vi "equilibrium_measurements_autofocus_build.vi"() -> ()   [LabVIEW 2019]
uses:
  <vilib>/userDefined/High Color/IMAQdx.ctl
  <vilib>/vision/driver/IMAQdx.llb/IMAQdx Attribute Type.ctl
  <vilib>/vision/Management.llb/Cast Image 2 Method.ctl
  <vilib>/DAQmx/write.llb/DAQmx Write (Analog DBL 1Chan 1Samp).vi
  <vilib>/DAQmx/write.llb/DAQmx Write (Digital Bool 1Line 1Point).vi
  <vilib>/DAQmx/read.llb/DAQmx Read (Analog DBL 1Chan 1Samp).vi
  <vilib>/Analysis/baseanly.llb/Mean (DBL).vi
  <vilib>/DAQmx/create/channels.llb/DAQmx Create Channel (AO-Voltage-Basic).vi
  <vilib>/DAQmx/miscellaneous.llb/DAQmx Fill In Error Info.vi
  <vilib>/DAQmx/create/channels.llb/DAQmx Create Channel (AI-Temperature-Thermocouple).vi
  <vilib>/DAQmx/create/channels.llb/DAQmx Create Channel (DO-Digital Output).vi
  <vilib>/DAQmx/create/channels.llb/DAQmx Create Channel (CO-Pulse Generation-Frequency).vi
  <vilib>/DAQmx/configure/timing.llb/DAQmx Timing (Implicit).vi
  <vilib>/vision/driver/NI_Vision_Acquisition_Software.lvlib
  <resource>/objmgr/imaqdx.rc
  <vilib>/vision/NI_Vision_Development_Module.lvlib
  <vilib>/Analysis/NI_AALBase.lvlib
  <resource>/objmgr/daqmx.rc
panel:
  out "x-y":dbl
  out "Waveform Chart":dynamicdata(graph)
  out "Autofocus":bool
  out "Turn":bool
  out "displacement":i32
  out "steps":i32=1000
  out "Direction":bool
  in  "Direction Line":tag="Dev3/port1/line4"
  in  "Enable Drive":bool
  in  "Enable Line":tag="Dev3/port1/line1"
  in  "Step Signal \nOutput Line":tag="/Dev3/PFI2"
  in  "Step Pulse Train \nFrequency (Hz)":dbl=200.0 format="%.6f"
  out "Video":bool
  in  "Action":i32(listbox)
  out "meanIntensity":dbl[](array[numeric])
  out "varLaplacian":dbl[](array[numeric])
  out "mean":dbl
  out "variance":dbl
  out "Avg Intensity":dbl(graph)=4.716017316017316
  in  "Activate":bool
  out "Var of Laplacian":dbl(graph)=701.3672509340029
  in  "ROI":T1={"Global Rectangle"=[], "Contours"=[{"Contour Type"=0, "ROI Type"=3, "Points"=[231, 86, 235, 90]}, {"Contour Type"=0, "ROI Type"=3, "Points"=[193, 50, 270, 125]}]}
  in  "error in":errorcluster
  in  "File path for video":string="C:\\Users\\Aniket\\Desktop\\mCherry_calibration\\new_lens\\laser_calibration\\laser_and_heating\\"
  in  "Laser profile file path":path=path "C:/Users/Aniket/Desktop/mCherry_calibration/new_lens/laser_calibration/laser_profiles/new_profile.txt"
  in  "Trigger Laser":bool
  in  "Power Generator":refnum<visa-resource-name>="COM3"
  in  "Desired \nTemperature":dbl=20.0 format="%#_13g"
  in  "PID Control":bool
  in  "Image file path \n(Do not add specify file extension - set to png)":path=path "C:/Users/Aniket/Desktop/mCherry_calibration/new_lens/laser_calibration/laser_profiles.txt"
  out "Current \nTemperature":dbl format="%0.2f"
  out "?":dbl[](graph)=[37.63236695538445]
  out "error out 7":errorcluster
  out "error out 6":errorcluster
  out "error out 5":errorcluster
  out "Exposure Time":dbl
  in  "ON/OFF":bool
  out "error out 3":errorcluster
  in  "LED":dbl(slide) scale=0.0..10.0
  in  "Refresh":bool
  out "Record":bool
  out "Processed Frames per Second":dbl
  out "Acquired Frame Rate":dbl
  out "error out":errorcluster
  out "Camera Display":T2(plugin-control) caption="Image Out"
  in  "Frame Rate":dbl=20.0
  out "Attribute Information Array":T4(array[cluster])
  in  "Session In":T5="cam0"
  # "Spot motion"
  # "Stage motion"
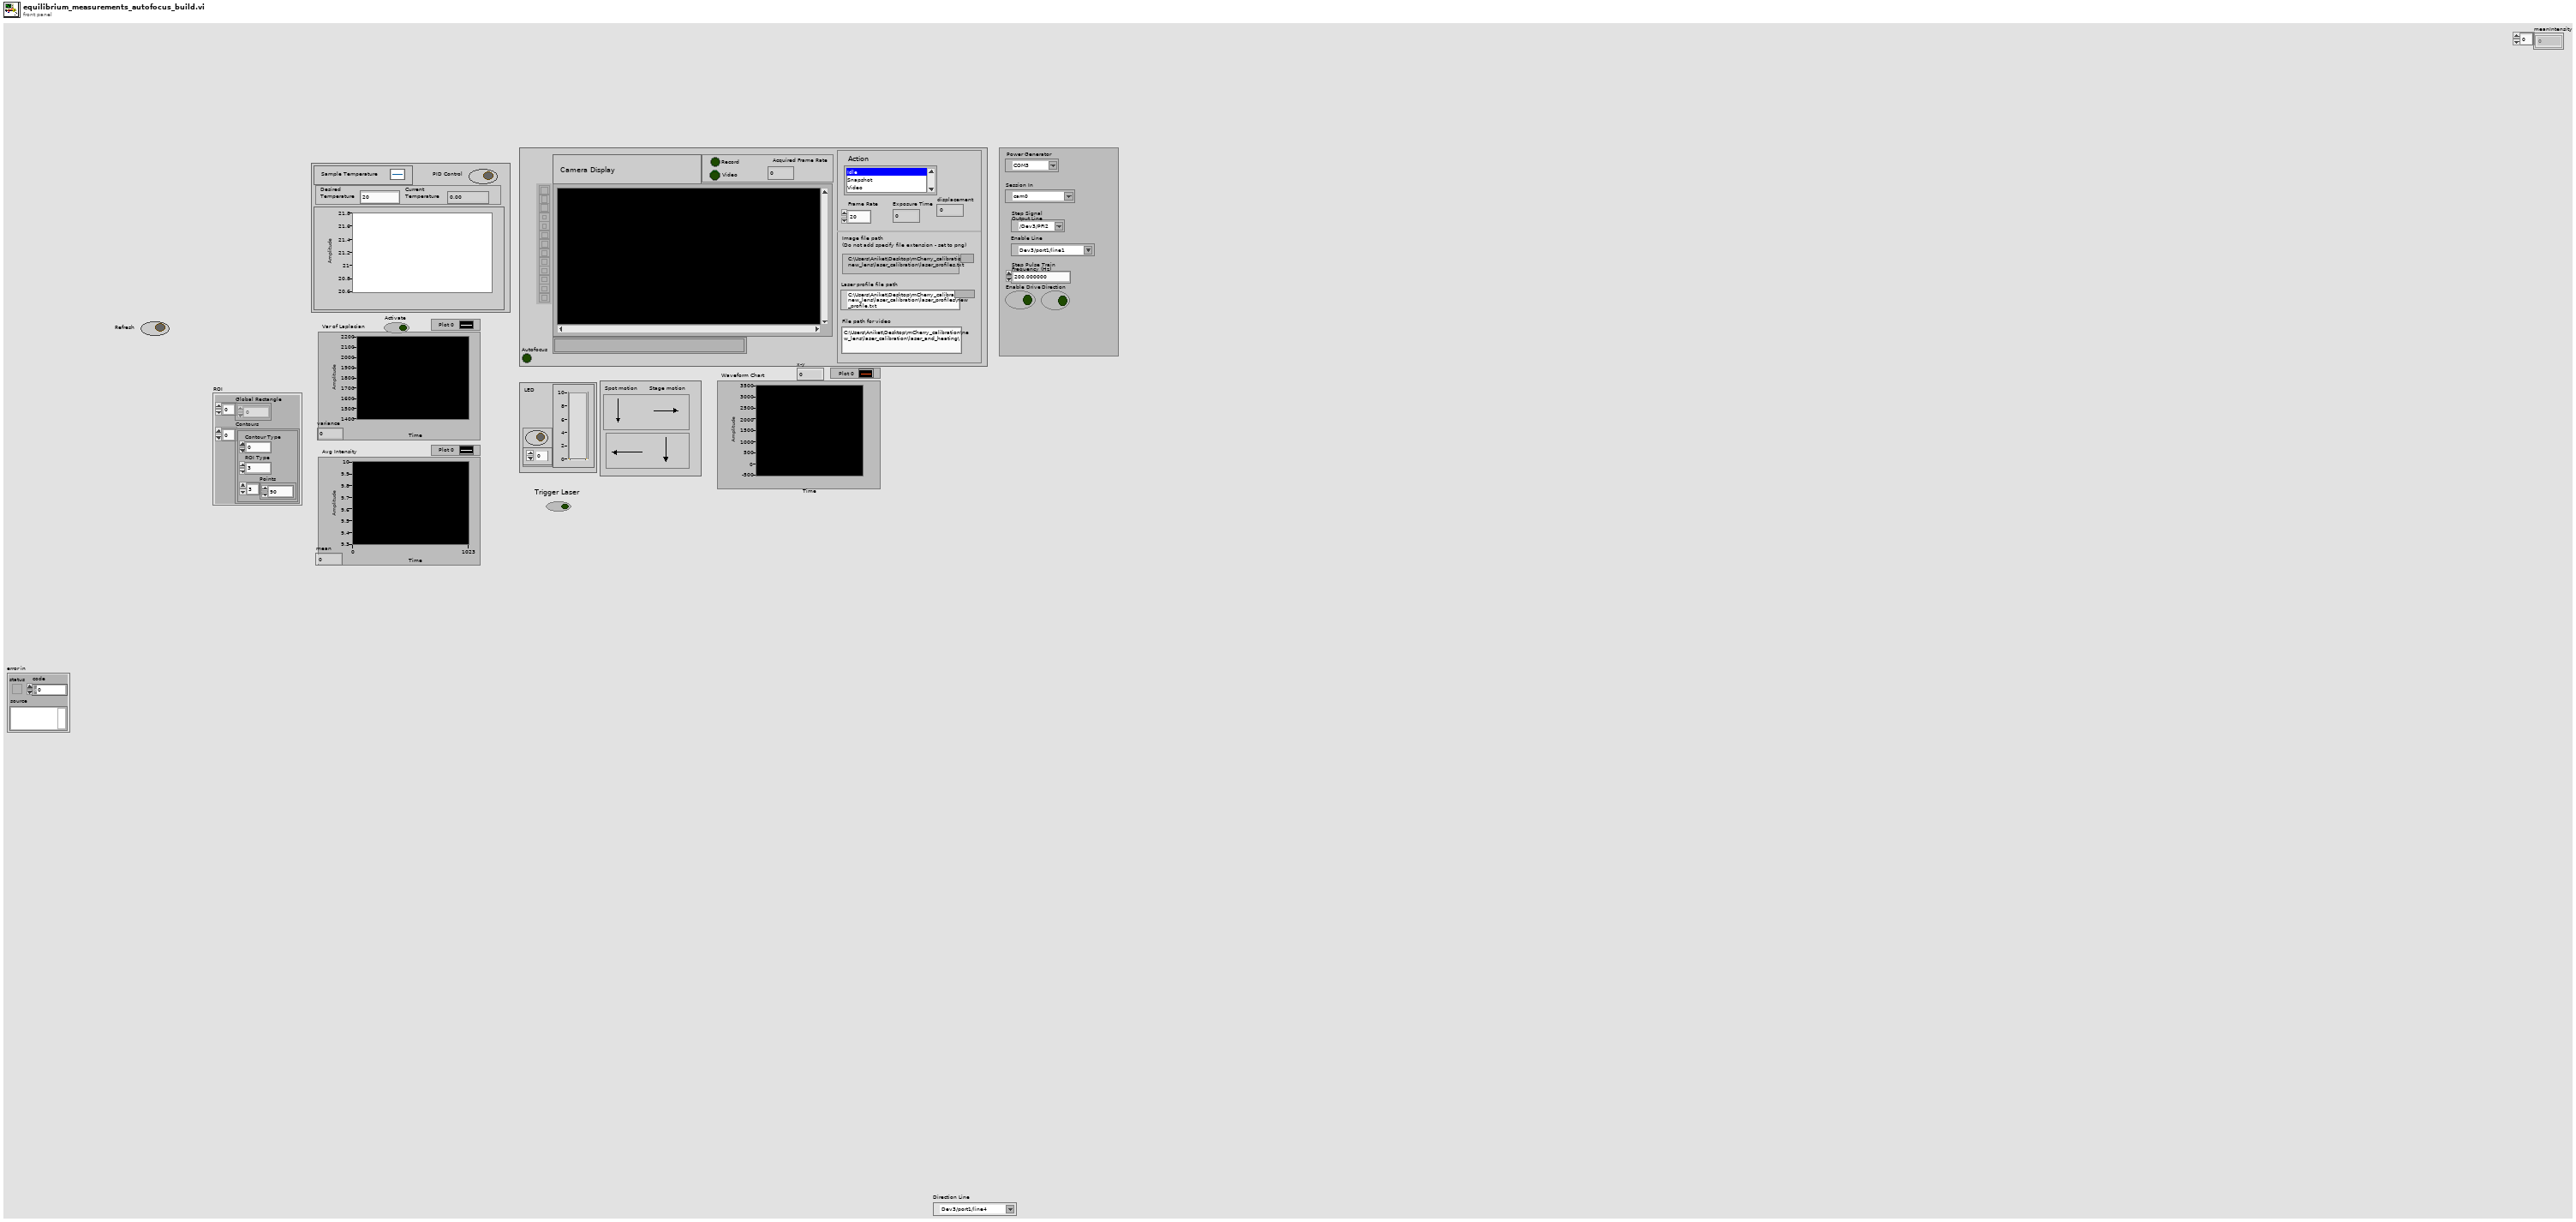
[diagram p1: front panel]
types:
  T1 = cluster{"Global Rectangle":i32[], "Contours":cluster{"Contour Type":u32, "ROI Type":u32, "Points":i32[]}[]}
  T2 = typedef "IMAQ Image.ctl" = refnum<image>
  T3 = typedef "NI_Vision_Acquisition_Software.lvlib/IMAQdx Attribute Type.ctl" = enum32{"U32", "I64", "DBL", "String", "Enum", "Bool", "Command"}
  T4 = cluster{"Attribute Type":T3, "Readable":bool, "Writable":bool, "Attribute Name":string}[]
  T5 = typedef "IMAQdx.ctl" = refnum<k21>
  T6 = typedef "Image Type" = u32
  T7 = typedef "ROI Descriptor" = cluster{"Global Rectangle":i32[], "Contours":cluster{"ID":enum32{"External", "Internal"}, "Type":u32, "Coordinates":i32[]}[]}
  T8 = typedef "IMAQ Rectangle" = cluster{"Left":i32, "Top":i32, "Right":i32, "Bottom":i32, "Rotation":dbl}
  T9 = cluster{"Mean Intensity":sgl, "Standard  Deviation":sgl, "Minimum Intensity":sgl, "Maximum Intensity":sgl}
  T10 = typedef "Cast Image 2 Method.ctl" = u32
  T11 = typedef "IMAQ AVI2 Refnum.ctl" = refnum<k20>
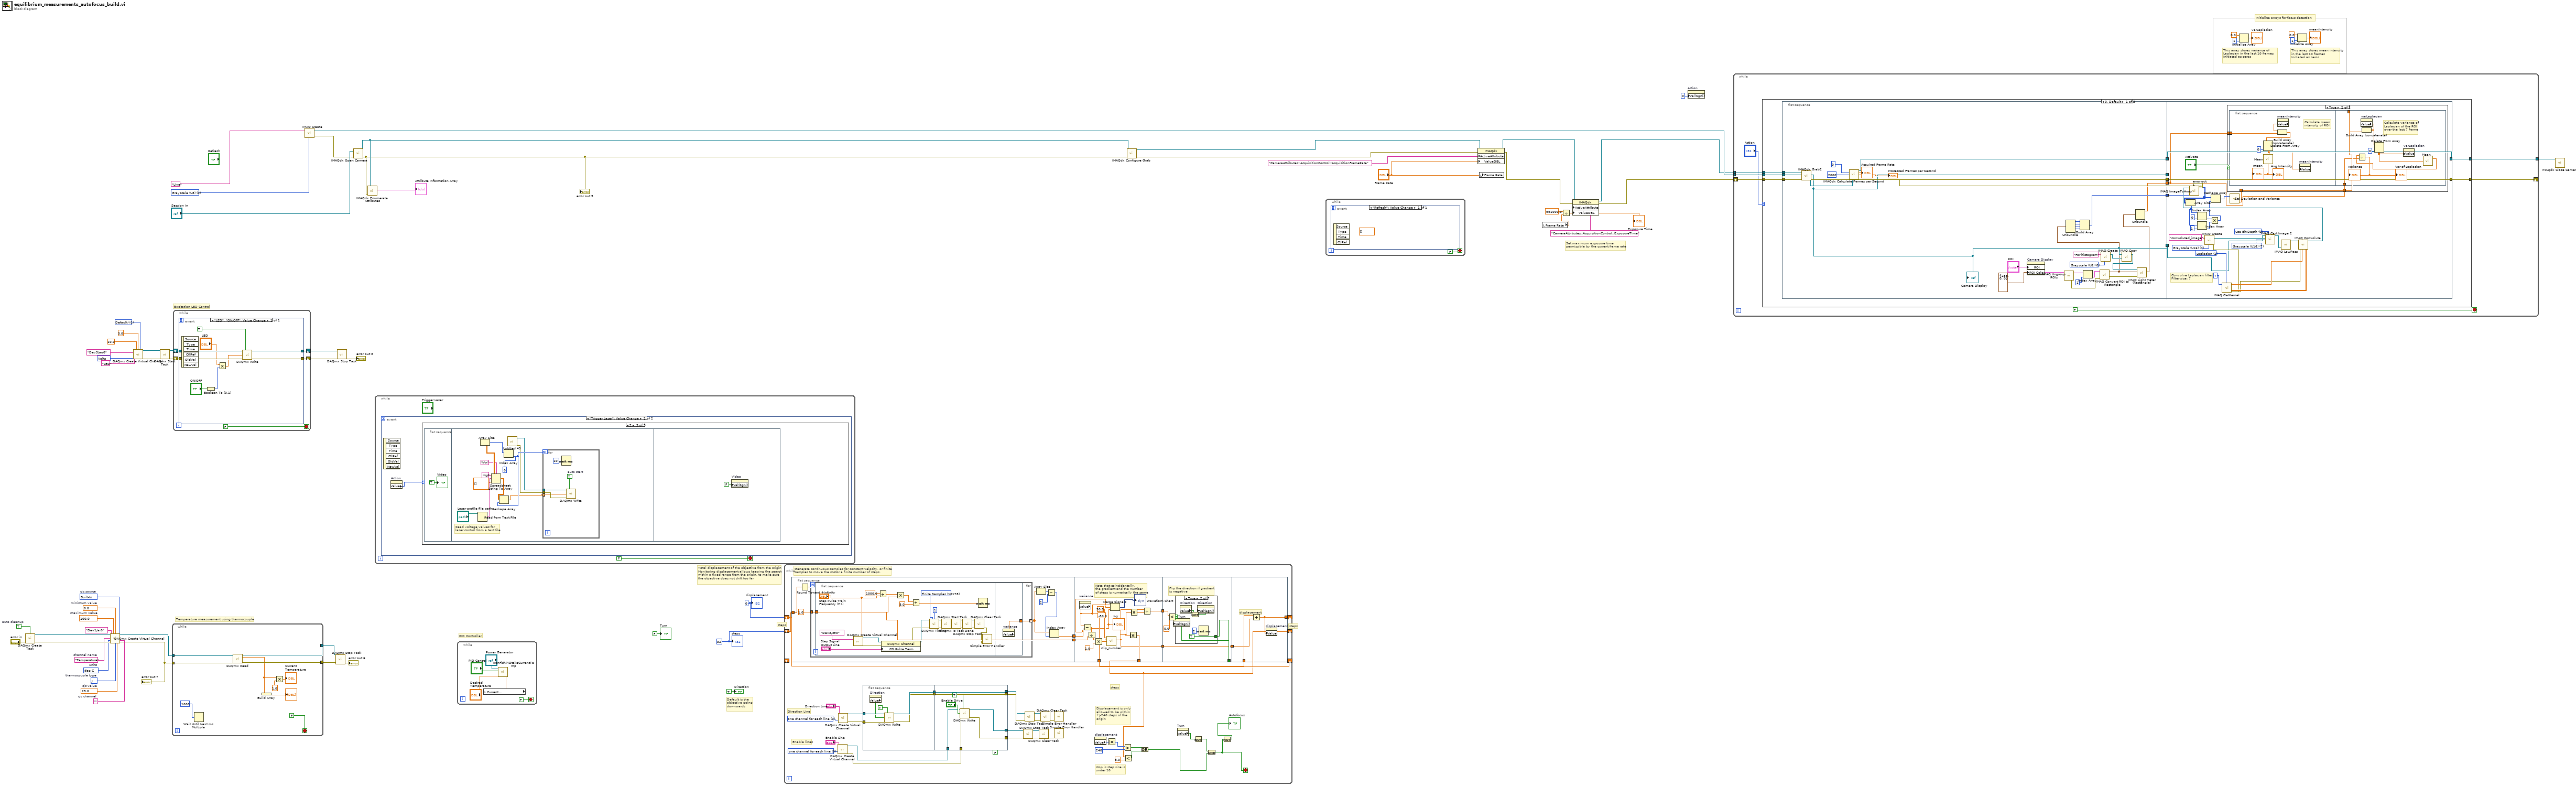
[diagram p0: block diagram]
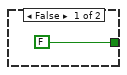
[diagram p2: hidden frame]
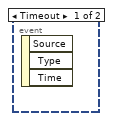
[diagram p3: hidden frame]
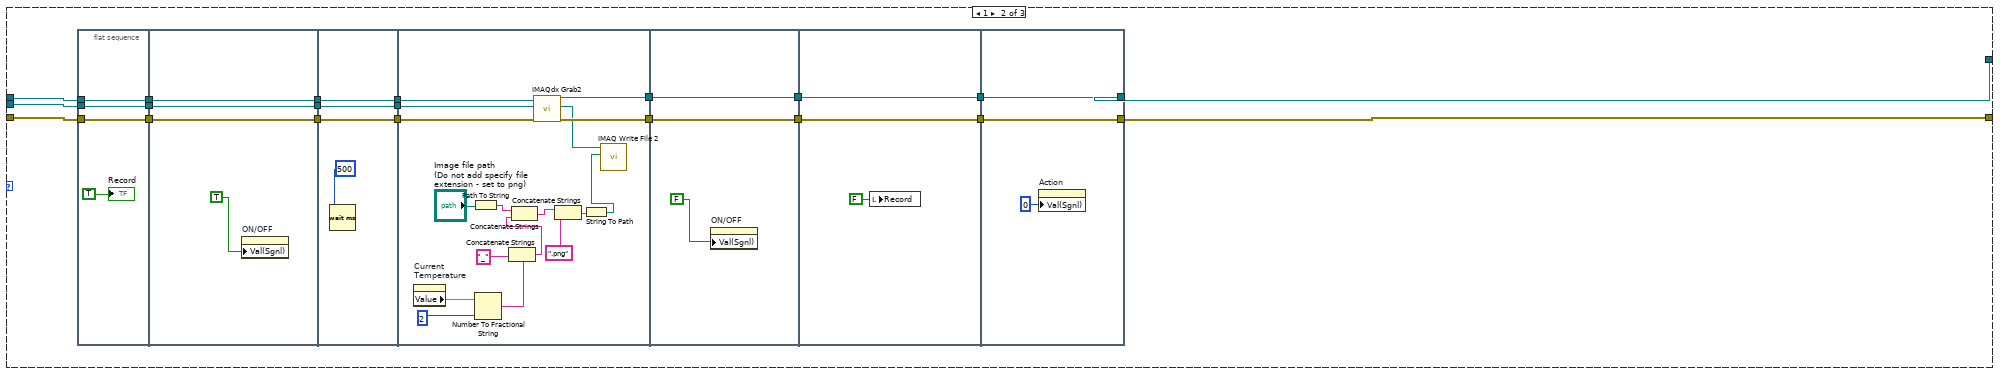
[diagram p7: hidden frame]
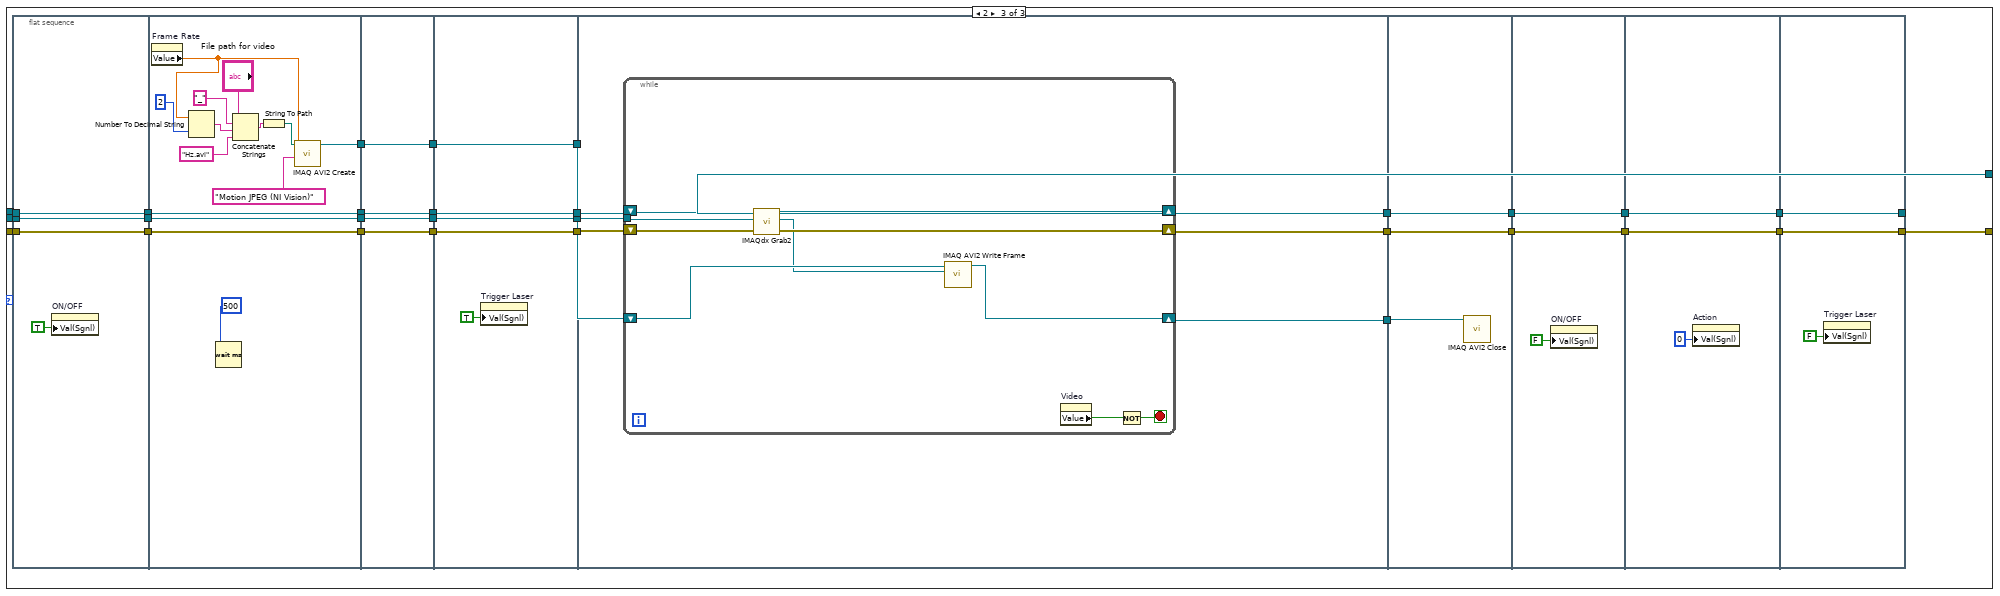
[diagram p8: hidden frame]
diagram:
  w4 = 0
  w3 = 32 ("samples per channel")
  w16 = 10200 items=["Built-In"=10200, "Constant Value"=10116, "Channel"=10113]  # cjc source
  w18 = ""  # cjc channel
  w19 = 25.0  # cjc value
  w20 = 10072 items=["J"=10072, "K"=10073, "N"=10077, "R"=10082, "S"=10085, "T"=10086, "B"=10047, "E"=10055]  # thermocouple type
  w21 = 10143 items=["deg C"=10143, "deg F"=10144, "Kelvins"=10325, "deg R"=10145, "From Custom Scale"=10065]  # units
  w17 = "Temperature"  # channel name
  w22 = 0.0  # minimum value
  w23 = 100.0  # maximum value
  w25 = TRUE  # auto cleanup
  w48 = 10348 items=["Volts"=10348, "From Custom Scale"=10065] ("units")
  w50 = -1 items=["Default"=-1, "RSE"=10083, "NRSE"=10078, "Differential"=10106, "Pseudodifferential"=12529] ("input terminal configuration")
  w62 = T6 0 items=["Grayscale (U8)", "Grayscale (I16)", "Grayscale (SGL)", "Complex (CSG)", "RGB (U32)", "HSL (U32)", "RGB (U64)", "Grayscale (U16)"] ("Image Type")
  # "Default is the\nobjective going\ndownwards"
  # "displacement"
  # "steps"
  # "steps"
  # "Total displacement of the objective from the origin\nMonitoring displacement allows keeping the search\nwithin a fixed range from the origin, to make sure\nthe objective does not drift too far"
  # "Set maximum exposure time \npermissible by the current frame rate"
  # "Excitation LED Control"
  # "Temperature measurement using thermocouple"
  # "PID Controller"
  # "Initialize arrays for focus detection"
  # "This array stores mean intensity in the last 10 frames\nInitiated as zeros"
  # "This array stores variance of Laplacian in the last 10 frames\nInitiated as zeros"
  n1 = call <vilib>:"DAQmx Create Task.vi"("auto cleanup"=w25, "error in"="error in") -> ("task out"=w24:refnum<k21>, "error out"=w26:errorcluster)  [unwired: 12 in]
  n2 = call-poly <vilib>:"DAQmx Create Virtual Channel.vi"("task in"=w24, "maximum value"=w23, "minimum value"=w22, "physical channels"=tag "Dev1/ai0", "cjc source"=w16, "name to assign"=w17, "units"=w21, "cjc channel"=w18, "error in"=w26, "thermocouple type"=w20, "cjc value"=w19) -> ("task out"=w15:refnum<k21>, "error out"=w14:errorcluster)  [unwired: 3 in]
  "error out 7" <- w14
  n3 = call-poly <vilib>:"DAQmx Create Virtual Channel.vi"("maximum value"=10.0, "minimum value"=0.0, "output terminal configuration"=w50, "physical channels"=tag "Dev3/ao0", "name to assign"="LED", "units"=w48) -> ("task out"=w46:refnum<k21>, "error out"=w45:errorcluster)  [unwired: 8 in]
  n4 = call <vilib>:"DAQmx Start Task.vi"("task/channels in"=w46, "error in"=w45) -> ("task out"=w44:refnum<k21>, "error out"=w43:errorcluster)  [unwired: 12 in]
  n5 = while {
    tunnel: w15 -> [w73]
    tunnel: w14 -> [w72]
    tunnel: [w71] -> w30
    tunnel: [w70] -> w29
    stop <- FALSE ("Monitor Temperature") stop-if-true
    n6 = Wait Until Next ms Multiple(millisecond multiple=u32 1000 ("millisecond timer value")) -> ()  [unwired: 1 out]
    n7 = call-poly <vilib>:"DAQmx Read.vi"("task/channels in"=w73, "error in"=w72) -> ("task out"=w71:refnum<k21>, "data"=w66:dbl, "error out"=w70:errorcluster)  [unwired: 11 in]
    n8 = Build Array(w66) -> (→"?":dbl[])
    n9 = Multiply(x=w66, y=1.0) -> (x*y=→"Current \nTemperature":dbl)
  }
  n10 = while {
    shift-right: [w77] -> w42
    shift-left: w44 -> [w79]
    shift-right: [w76] -> w41
    shift-left: w43 -> [w78]
    stop <- FALSE stop-if-true
    n11 = event shown="[0] \"LED\", \"ON/OFF\": Value Change" {
      selector: _ -> [_]
      dyn-events: _ -> [_]
      timeout: _ -> [_]
      tunnel: w79 -> [w88]
      tunnel: w78 -> [w87]
      tunnel: [w86] -> w77
      tunnel: [w85] -> w76
      event "LED", "ON/OFF": Value Change {
        n12 = event-data() -> ()  [unwired: 1 in, 6 out]
        n13 = Boolean To (0,1)(Boolean="ON/OFF") -> (0, 1=w81:i16)
        n14 = Multiply(x="LED", y=w81) -> (x*y=w80:dbl)
        n15 = call-poly <vilib>:"DAQmx Write.vi"("task/channels in"=w88, "auto start"=TRUE, "data"=w80, "error in"=w87) -> ("task out"=w86:refnum<k21>, "error out"=w85:errorcluster)  [unwired: 9 in, 1 out]
      }
    }
  }
  n16 = call "IMAQ Create"("Image Name"="Live", "Image Type"=w62) -> ("New Image"=w56:T2, "error out"=w55:errorcluster)  [unwired: 3 in]
  n17 = call <vilib>:"DAQmx Stop Task.vi"("task/channels in"=w30, "error in"=w29) -> ("error out"=→"error out 6":errorcluster)  [unwired: 12 in, 1 out]
  n18 = call <vilib>:"DAQmx Stop Task.vi"("task/channels in"=w42, "error in"=w41) -> ("error out"=→"error out 3":errorcluster)  [unwired: 12 in, 1 out]
  n19 = call <vilib>:"IMAQdx Open Camera.vi"("error in"=w55, "Session In"="Session In") -> ("error out"=w60:errorcluster, "Session Out"=w61:T5)  [unwired: 8 in]
  "error out 5" <- w60
  n20 = call <vilib>:"IMAQdx Enumerate Attributes.vi"("error in"=w60, "Session In"=w61) -> ("Attribute Information Array"=→"Attribute Information Array":T4)  [unwired: 7 in, 2 out]
  n21 = while {
    stop <- FALSE stop-if-true
    n22 = event shown="[1] \"Trigger Laser\": Value Change" {
      selector: _ -> [_ _]
      dyn-events: _ -> [_ _]
      timeout: _ -> [_ _]
      event Timeout {
        n23 = event-data() -> ()  [unwired: 1 in, 3 out]
      }
      event "Trigger Laser": Value Change {
        n24 = event-data() -> ()  [unwired: 1 in, 6 out]
        n25 = property on="Action" class="LstBox (strict)"() -> ("Value"=w90:i32)  [unwired: 2 in, 2 out]
        n26 = case shown="2" w90 {
          frame 0, Default {
          }
          frame 1 {
          }
          frame 2 {
            n27 = flat-sequence {
              frame #0 {
                "Video" <- TRUE ("Video")
              }
              frame #1 {
                # "Read voltage values for\nlaser control from a text file"
                n28 = Read from Text File(file (use dialog)="Laser profile file path") -> (text=w99:string)  [unwired: 3 in, 3 out]
                n29 = Spreadsheet String To Array(delimiter (Tab)="\r\n", format string="%f", spreadsheet string=w99, array type (2D Dbl)=dbl[][] []) -> (array=w101:dbl[][])
                n30 = Array Size(array=w101) -> (size(s)=w100:i32[])
                n31 = Index Array(array=w100, index=0) -> (element=w103:i32)
                n32 = Reshape Array(w101, w103) -> (w102:dbl[])
                n33 = call "Untitled 43.vi"() -> ("error out"=w92:errorcluster, "task out"=w93:refnum<k21>)  [unwired: 10 in]
                n34 = for {
                  N: w103 -> [_]
                  tunnel: w102 -> [w104] mode=indexing
                  tunnel: w93 -> [w106]
                  tunnel: w92 -> [w105]
                  w107 = TRUE  # auto start
                  n35 = Wait (ms)(milliseconds to wait=u32 10) -> ()  [unwired: 1 out]
                  n36 = call-poly <vilib>:"DAQmx Write.vi"("task/channels in"=w106, "auto start"=w107, "data"=w104, "error in"=w105) -> ()  [unwired: 9 in, 3 out]
                }
              }
              frame #2 {
                n37 = property on="Video" class="Bool (strict)"("Val(Sgnl)"=FALSE ("Value (Signaling)")) -> ()  [unwired: 2 in, 2 out]
              }
            }
          }
        }
      }
    }
  }
  n38 = while {
    stop <- FALSE stop-if-true
    n39 = local read "Current \nTemperature"() -> (w113:dbl)
    n40 = call "IronFishPIDtakeCurrentTemp.vi"(0:"Power Generator", "Switch"="PID Control", "Desired Temp"="Desired \nTemperature", "Current Temp"=w113) -> ()  [unwired: 4 in, 1 out]
  }
  n41 = while {
    shift-right: [w136] -> _
    shift-left: _ -> [_]
    shift-right: [w135] -> _
    shift-left: w4 -> [w134]
    shift-right: [w123] -> _
    shift-left: w3 -> [w133]
    stop <- w116 stop-if-true
    (unwired) FALSE
    w138 = 0 items=["one channel for each line", "one channel for all lines"] ("line grouping")
    w137 = 0 items=["one channel for each line", "one channel for all lines"] ("line grouping")
    # "stop is step size is \nunder 10"
    # "steps"
    # "Displacement is only\nallowed to be within \n+/-240 steps of the\norigin"
    # "Direction Line"
    # "Enable lines"
    # "Generate continuous samples for constant velocity, or finite \nsamples to move the motor a finite number of steps."
    n42 = flat-sequence {
      tunnel: [w178] -> w132
      tunnel: w133 -> [w172]
      tunnel: [w173] -> w117
      tunnel: [w209] -> w136
      tunnel: [w216] -> w123
      tunnel: w132 -> [w219]
      tunnel: [w217] -> w124
      tunnel: [w215] -> w122
      tunnel: w117 -> [w208]
      tunnel: [w224] -> w125
      tunnel: w124 -> [w222]
      tunnel: w122 -> [w224]
      tunnel: [w220] -> w121
      tunnel: w125 -> [w232]
      tunnel: [w231] -> w135
      tunnel: w134 -> [w230]
      frame #0 {
        w178 = 1.0 ("samples per channel")
        n43 = Round Toward +Infinity(x=w172) -> (ceil(x): smallest int >= x=w171:dbl)
        n44 = for {
          N: w171 -> [_]
          tunnel: w178 -> [w180]
          tunnel: [w179] -> w177 mode=indexing
          n45 = flat-sequence {
            tunnel: w180 -> [w200]
            tunnel: [w205] -> w179
            frame #0 {
              w194 = 10178 items=["Finite Samples"=10178, "Continuous Samples"=10123, "Hardware Timed Single Point"=12522] ("sample mode")
              n46 = call-poly <vilib>:"DAQmx Create Virtual Channel.vi"("frequency"="Step Pulse Train \nFrequency (Hz)", "counter"=tag "Dev3/ctr0") -> ("task out"=w186:refnum<k21>, "error out"=w185:errorcluster)  [unwired: 12 in]
              n47 = Divide(x=1000.0, y="Step Pulse Train \nFrequency (Hz)") -> (x/y=w189:dbl)
              n48 = property class="DAQmx Channel"(reference=w186, error in=w185, "CO.Pulse.Term"="Step Signal \nOutput Line") -> (reference out=w193:refnum<k21>, error out=w192:errorcluster)
              n49 = Multiply(x=w189, y=w200) -> (x*y=w191:dbl)
              n50 = Add(x=w191, y=5.0) -> (x+y=w197:dbl)
              n51 = call-poly <vilib>:"DAQmx Timing.vi"("task/channels in"=w193, "sample mode"=w194, "samples per channel"=1, "error in"=w192) -> ("task out"=w196:refnum<k21>, "error out"=w195:errorcluster)  [unwired: 10 in]
              n52 = call <vilib>:"DAQmx Start Task.vi"("task/channels in"=w196, "error in"=w195) -> ("task out"=w199:refnum<k21>, "error out"=w198:errorcluster)  [unwired: 12 in]
              n53 = call <vilib>:"DAQmx Is Task Done.vi"("task/channels in"=w199, "error in"=w198) -> ("task out"=w203:refnum<k21>, "error out"=w202:errorcluster)  [unwired: 11 in, 1 out]
              n54 = call <vilib>:"DAQmx Stop Task.vi"("task/channels in"=w203, "error in"=w202) -> ("task out"=w204:refnum<k21>, "error out"=w201:errorcluster)  [unwired: 12 in]
              n55 = call <vilib>:"DAQmx Clear Task.vi"("task in"=w204, "error in"=w201) -> ("error out"=w181:errorcluster)  [unwired: 13 in]
              n56 = Wait (ms)(milliseconds to wait=w197) -> ()  [unwired: 1 out]
              n57 = call <vilib>:"Simple Error Handler.vi"("error in (no error)"=w181) -> ()  [unwired: 4 in, 5 out]
            }
            frame #1 {
              n58 = property on="variance" class="DigNum (strict)"() -> ("Value"=w205:dbl)  [unwired: 2 in, 2 out]
            }
          }
        }
        n59 = Array Size(array=w177) -> (size(s)=w176:i32)
        n60 = Subtract(x=w176, y=2) -> (x-y=w174:i32)
        n61 = Index Array(array=w177, index=w174) -> (element=w173:dbl)
      }
      frame #1 {
        # "Note that coincidentally,\nthe gradient and the number\nof steps is numerically the same"
        n62 = property on="variance" class="DigNum (strict)"() -> ("Value"=w209:dbl)  [unwired: 2 in, 2 out]
        n63 = Subtract(x=w209, y=w208) -> (x-y=w207:dbl)
        "x-y" <- w207
        n64 = Divide(x=w207, y=w219) -> (x/y=w211:dbl)
        n65 = Multiply(x=w211, y=1.0) -> (x*y=w212:dbl)
        n66 = call "clip_number.vi"("x"=w212, "lower limit"=-50.0, "upper limit"=50.0) -> ("x-y"=w215:dbl)  [unwired: 8 in]
        n67 = Merge Signals(w209, w208, w207) -> (→"Waveform Chart":dynamicdata)
        n68 = Absolute Value(x=w215) -> (abs(x)=w216:dbl)
        n69 = Absolute Value(x=w215) -> (abs(x)=w218:dbl)
        n70 = Divide(x=w215, y=w218) -> (x/y=w217:dbl)
      }
      frame #2 {
        # "Flip the direction if gradient\nis negative"
        n71 = Less?(x=w222, y=0.0) -> (x < y?=w223:bool)
        n72 = case shown="True" w223 {
          tunnel: [FALSE ("Value (Signaling)") TRUE ("Value (Signaling)")] -> w220
          frame False {
          }
          frame True {
            n73 = property on="Direction" class="Bool (strict)"() -> ("Value"=w229:bool)  [unwired: 2 in, 2 out]
            n74 = Not(x=w229) -> (.not. x?=w228:bool)
            n75 = property on="Direction" class="Bool (strict)"("Val(Sgnl)"=w228) -> ()  [unwired: 2 in, 2 out]
            n76 = Wait (ms)(milliseconds to wait=u32 2) -> ()  [unwired: 1 out]
          }
        }
      }
      frame #3 {
        n77 = Add(x=w230, y=w232) -> (x+y=w231:dbl)
        n78 = property on="displacement" class="DigNum (strict)"("Value"=w231) -> ()  [unwired: 2 in, 2 out]
      }
    }
    n79 = call-poly <vilib>:"DAQmx Create Virtual Channel.vi"("lines"="Enable Line", "line grouping"=w137) -> ("task out"=w151:refnum<k21>, "error out"=w152:errorcluster)  [unwired: 12 in]
    n80 = call-poly <vilib>:"DAQmx Create Virtual Channel.vi"("lines"="Direction Line", "line grouping"=w138) -> ("task out"=w147:refnum<k21>, "error out"=w148:errorcluster)  [unwired: 12 in]
    n81 = flat-sequence {
      tunnel: w147 -> [w161]
      tunnel: w148 -> [w160]
      tunnel: [w159] -> w156
      tunnel: [w158] -> w155
      tunnel: [w169] -> w150
      tunnel: [w170] -> w149
      tunnel: w156 -> [w170]
      tunnel: w155 -> [w169]
      tunnel: w151 -> [w166]
      tunnel: w152 -> [w165]
      tunnel: [w164] -> w153
      tunnel: [w163] -> w154
      frame #0 {
        n82 = property on="Direction" class="Bool (strict)"() -> ("Value"=w157:bool)  [unwired: 2 in, 2 out]
        n83 = call-poly <vilib>:"DAQmx Write.vi"("task/channels in"=w161, "auto start"=TRUE, "data"=w157, "error in"=w160) -> ("task out"=w159:refnum<k21>, "error out"=w158:errorcluster)  [unwired: 9 in, 1 out]
      }
      frame #1 {
        n84 = call-poly <vilib>:"DAQmx Write.vi"("task/channels in"=w166, "auto start"=TRUE, "data"="Enable Drive", "error in"=w165) -> ("task out"=w164:refnum<k21>, "error out"=w163:errorcluster)  [unwired: 9 in, 1 out]
      }
    }
    n85 = call <vilib>:"DAQmx Stop Task.vi"("task/channels in"=w153, "error in"=w154) -> ("task out"=w140:refnum<k21>, "error out"=w141:errorcluster)  [unwired: 12 in]
    n86 = call <vilib>:"DAQmx Stop Task.vi"("task/channels in"=w149, "error in"=w150) -> ("task out"=w146:refnum<k21>, "error out"=w145:errorcluster)  [unwired: 12 in]
    n87 = call <vilib>:"DAQmx Clear Task.vi"("task in"=w140, "error in"=w141) -> ("error out"=w142:errorcluster)  [unwired: 13 in]
    n88 = call <vilib>:"DAQmx Clear Task.vi"("task in"=w146, "error in"=w145) -> ("error out"=w144:errorcluster)  [unwired: 13 in]
    n89 = call <vilib>:"Simple Error Handler.vi"("error in (no error)"=w144) -> ()  [unwired: 4 in, 5 out]
    n90 = call <vilib>:"Simple Error Handler.vi"("error in (no error)"=w142) -> ()  [unwired: 4 in, 5 out]
    n91 = property on="displacement" class="DigNum (strict)"() -> ("Value"=w130:i32)  [unwired: 2 in, 2 out]
    n92 = Absolute Value(x=w130) -> (abs(x)=w129:i32)
    n93 = Greater?(x=w129, y=240) -> (0:w128:bool)
    n94 = Less?(x=w123, y=8.0) -> (x < y?=w127:bool)
    n95 = Or(x=w128, y=w127) -> (x .or. y?=w118:bool)
    n96 = property on="Turn" class="Bool (strict)"("Val(Sgnl)"=w121) -> ()  [unwired: 2 in, 2 out]
    n97 = property on="Turn" class="Bool (strict)"() -> ("Value"=w120:bool)  [unwired: 2 in, 2 out]
    n98 = Not(x=w120) -> (.not. x?=w119:bool)
    n99 = And(x=w119, y=w118) -> (x .and. y?=w116:bool)
    n100 = Not(x=w116) -> (.not. x?=→"Autofocus":bool)
  }
  n101 = call <vilib>:"IMAQdx Configure Grab.vi"("error in"=w60, "Session In"=w61) -> ("error out"=w58:errorcluster, "Session Out"=w39:T5)  [unwired: 8 in]
  n102 = while {
    stop <- FALSE stop-if-true
    n103 = event shown="[0] \"Refresh\": Value Change" {
      selector: _ -> [_]
      dyn-events: _ -> [_]
      timeout: _ -> [_]
      event "Refresh": Value Change {
        (unwired) dbl[] [] ("History Data")
        n104 = event-data() -> ()  [unwired: 1 in, 4 out]
      }
    }
  }
  n105 = property class="IMAQdx"(reference=w39, error in=w58, "ActiveAttribute"="CameraAttributes::AcquisitionControl::AcquisitionFrameRate", "ValueDBL"="Frame Rate") -> (reference out=w34:T5, error out=w32:errorcluster)
  n106 = local write "Frame Rate"("Frame Rate") -> ()
  n107 = local read "Frame Rate"() -> (w36:dbl)
  n108 = Divide(x=991000.0, y=w36) -> (x/y=w35:dbl)
  "Exposure Time" <- w35
  n109 = property class="IMAQdx"(reference=w34, error in=w32, "ActiveAttribute"="CameraAttributes::AcquisitionControl::ExposureTime", "ValueDBL"=w35) -> (reference out=w33:T5, error out=w31:errorcluster)
  n110 = property on="Action" class="LstBox (strict)"("Val(Sgnl)"=0 ("Value (Signaling)")) -> ()  [unwired: 2 in, 2 out]
  n111 = while {
    tunnel: w33 -> [w240]
    tunnel: w56 -> [w238]
    shift-right: [w237] -> w54
    shift-left: w31 -> [w239]
    tunnel: [w234] -> w6
    stop <- FALSE ("Stop") stop-if-true
    n112 = case shown="0, Default" "Action" {
      tunnel: w240 -> [w251 w343 w414]
      tunnel: w239 -> [w250 w345 w412]
      tunnel: w238 -> [w249 w344 w413]
      tunnel: [w248 w346 w410] -> w237
      tunnel: [w247 w347 w411] -> w234
      frame 0, Default {
        n113 = flat-sequence {
          tunnel: w251 -> [w281]
          tunnel: w250 -> [w280]
          tunnel: w249 -> [w279]
          tunnel: [w278] -> w246
          tunnel: [w276] -> w245
          tunnel: [w263] -> w244
          tunnel: [w263] -> w243
          tunnel: [w255] -> w242
          tunnel: [w252] -> w241
          tunnel: [w309] -> w247
          tunnel: [w310] -> w248
          tunnel: w246 -> [w310]
          tunnel: w245 -> [w309]
          tunnel: w244 -> [_]
          tunnel: w243 -> [w291]
          tunnel: w242 -> [w300]
          tunnel: w241 -> [w282]
          frame #0 {
            w264 = T6 0 items=["Grayscale (U8)", "Grayscale (I16)", "Grayscale (SGL)", "Complex (CSG)", "RGB (U32)", "HSL (U32)", "RGB (U64)", "Grayscale (U16)"] ("Image Type")
            n114 = call <vilib>:"IMAQdx Grab2.vi"("error in"=w280, "Image In"=w279, "Session In"=w281) -> ("error out"=w278:errorcluster, "Image Out"=w263:T2, "Session Out"=w277:T5)  [unwired: 5 in, 1 out]
            "Camera Display" <- w263
            n115 = call <vilib>:"IMAQdx Calculate Frames per Second.vi"("Session In"=w277, "Buffer Number"=u32 0, "Minimum Display Update Interval (ms)"=u32 2000) -> ("Session Out"=w276:T5, "Acquired Frames per Second"=→"Acquired Frame Rate":dbl, "Processed Frames per Second"=→"Processed Frames per Second":dbl)  [unwired: 6 in, 4 out]
            n116 = property on="Camera Display" class="ImageControl"("ROI"="ROI", "ROI Color"=cluster{"Red":u8, "Green":u8, "Blue":u8} {"Red"=255, "Green"=0, "Blue"=0}) -> ()  [unwired: 2 in, 2 out]
            n117 = call "IMAQ Ungroup ROIs"("ROI Descriptor"="ROI") -> ("error out"=w267:errorcluster, "ROI Descriptors out"=w270:T7[])  [unwired: 3 in]
            n118 = Index Array(array=w270, index=1) -> (element=w268:T7)
            n119 = call "IMAQ Convert ROI to Rectangle"("error in (no error)"=w267, "ROI Descriptor"=w268) -> ("error out"=w266:errorcluster, "Rectangle"=w260:T8)  [unwired: 7 in]
            n120 = Unbundle(w260) -> ("Left"=w259:i32, "Top"=w258:i32, "Right"=w257:i32, "Bottom"=w256:i32)  [unwired: 1 out]
            n121 = Build Array(w259, w258, w257, w256) -> (w255:i32[])
            n122 = call "IMAQ Create"("Image Name"="For histogram", "Image Type"=w264) -> ("New Image"=w262:T2)  [unwired: 3 in, 1 out]
            n123 = call "IMAQ Copy"("Image Dst"=w262, "Image Src"=w263) -> ("Image Dst Out"=w261:T2)  [unwired: 4 in, 1 out]
            n124 = call "IMAQ Light Meter (Rectangle)"("error in (no error)"=w266, "Rectangle"=w260, "Image"=w261) -> ("Gray Level Intensities"=w253:T9)  [unwired: 4 in, 4 out]
            n125 = Unbundle(w253) -> ("Mean Intensity"=w252:sgl)  [unwired: 3 out]
          }
          frame #1 {
            w287 = T6 7 items=["Grayscale (U8)", "Grayscale (I16)", "Grayscale (SGL)", "Complex (CSG)", "RGB (U32)", "HSL (U32)", "RGB (U64)", "Grayscale (U16)"] ("Image Type")
            w290 = T10 0 items=["Use Bit Depth", "Shift", "Use Lookup Table"] ("Method")
            w305 = u16 2 items=["Gradient"=1, "Laplacian"=2, "Smoothing"=3, "Gaussian"=4] ("Kernel Family")
            w307 = T6 7 items=["Grayscale (U8)", "Grayscale (I16)", "Grayscale (SGL)", "Complex (CSG)", "RGB (U32)", "HSL (U32)", "RGB (U64)", "Grayscale (U16)"] ("Image Type")
            # "Convolve Laplacian filter \nFilter size: 7"
            n126 = call "IMAQ Create"("Image Name"="convoluted_image", "Image Type"=w307) -> ("New Image"=w289:T2, "error out"=w301:errorcluster)  [unwired: 3 in]
            n127 = call "IMAQ GetKernel"("Kernel Family"=w305, "error in (no error)"=w301, "Kernel Size (3,5,...)"=7) -> ("error out"=w302:errorcluster, "Kernel"=w303:sgl[][], "Divider"=w304:sgl)  [unwired: 5 in, 1 out]
            n128 = call "IMAQ Cast Image 2"("Image Src"=w291, "Method"=w290, "Image Dst"=w289, "Image Type"=w287) -> ("Image Dst Out"=w288:T2)  [unwired: 10 in, 1 out]
            n129 = call "IMAQ LowPass"("Image Src"=w288) -> ("Image Dst Out"=w292:T2)  [unwired: 6 in, 1 out]
            n130 = call "IMAQ Convolute"("Kernel"=w303, "Divider (kernel sum)"=w304, "error in (no error)"=w302, "Image Src"=w292) -> ("Image Dst Out"=w299:T2)  [unwired: 6 in, 1 out]
            n131 = call "IMAQ ImageToArray"("Optional Rectangle"=w300, "Image"=w299) -> ("Image Pixels (U16)"=w283:u16[][])  [unwired: 2 in, 4 out]
            n132 = Array Size(array=w283) -> (size(s)=w286:i32[])
            n133 = Index Array(array=w286, index=0 ("index (row)")) -> (element=w296:i32)
            n134 = Index Array(array=w286, index=1) -> (element=w295:i32)
            n135 = Multiply(x=w296, y=w295) -> (x*y=w285:i32)
            n136 = Reshape Array(w283, w285) -> (w284:u16[])
            n137 = call <vilib>:"Std Deviation and Variance.vi"("X"=w284) -> ("variance"=w293:dbl)  [unwired: 1 in, 2 out]
            n138 = case shown="True" "Activate" {
              tunnel: w293 -> [_ w313]
              tunnel: w282 -> [_ w312]
              tunnel: w282 -> [_ w311]
              frame False {
              }
              frame True {
                n139 = flat-sequence {
                  tunnel: w311 -> [w314]
                  tunnel: w313 -> [w323]
                  tunnel: w312 -> [w327]
                  frame #0 {
                    # "Calculate mean \nintensity of ROI"
                    n140 = property on="meanIntensity" class="Arr (strict)"() -> ("Value"=w317:dbl[])  [unwired: 2 in, 2 out]
                    n141 = Build Array (concatenate)(w317, w314) -> (w316:dbl[])
                    n142 = Delete From Array(array=w316, index=0) -> (array with subset deleted=w315:dbl[])  [unwired: 1 in, 1 out]
                    n143 = call-poly <vilib>:"Mean.vi"("X"=w315) -> ("mean"=→"Avg Intensity" →"mean":dbl)  [unwired: 1 out]
                    n144 = property on="meanIntensity" class="Arr (strict)"("Value"=w315) -> ()  [unwired: 2 in, 2 out]
                  }
                  frame #1 {
                    # "Calculate variance of\nLaplacian of the ROI\nover the last 7 frame"
                    n145 = property on="varLaplacian" class="Arr (strict)"() -> ("Value"=w324:dbl[])  [unwired: 2 in, 2 out]
                    n146 = Build Array (concatenate)(w324, w323) -> (w322:dbl[])
                    n147 = Delete From Array(array=w322, index=0) -> (array with subset deleted=w321:dbl[])  [unwired: 1 in, 1 out]
                    n148 = property on="varLaplacian" class="Arr (strict)"("Value"=w321) -> ()  [unwired: 2 in, 2 out]
                    n149 = call-poly <vilib>:"Mean.vi"("X"=w321) -> ("mean"=w326:dbl)  [unwired: 1 out]
                    n150 = Divide(x=w326, y=w327) -> (x/y=→"Var of Laplacian" →"variance":dbl)
                  }
                }
              }
            }
          }
        }
      }
      frame 1 {
        n151 = flat-sequence {
          tunnel: w343 -> [w349]
          tunnel: w344 -> [w350]
          tunnel: w345 -> [w351]
          tunnel: [w351] -> w332
          tunnel: [w350] -> w331
          tunnel: [w349] -> w330
          tunnel: [w355] -> w338
          tunnel: [w354] -> w336
          tunnel: [w353] -> w334
          tunnel: w332 -> [w355]
          tunnel: w331 -> [w354]
          tunnel: w330 -> [w353]
          tunnel: w338 -> [w359]
          tunnel: [w359] -> w337
          tunnel: w336 -> [w358]
          tunnel: [w358] -> w335
          tunnel: w334 -> [w357]
          tunnel: [w357] -> w333
          tunnel: [w372] -> w342
          tunnel: [w376] -> w340
          tunnel: w337 -> [w375]
          tunnel: w335 -> [w374]
          tunnel: w333 -> [w373]
          tunnel: w342 -> [w379]
          tunnel: [w379] -> w341
          tunnel: w340 -> [w378]
          tunnel: [w378] -> w339
          tunnel: w341 -> [w382]
          tunnel: w339 -> [w381]
          tunnel: [w382] -> w329
          tunnel: [w381] -> w328
          tunnel: [w384] -> w346
          tunnel: [w385] -> w347
          tunnel: w329 -> [w385]
          tunnel: w328 -> [w384]
          frame #0 {
            "Record" <- TRUE ("Record")
          }
          frame #1 {
            n152 = property on="ON/OFF" class="Bool (strict)"("Val(Sgnl)"=TRUE ("ON/OFF")) -> ()  [unwired: 2 in, 2 out]
          }
          frame #2 {
            n153 = Wait (ms)(milliseconds to wait=u32 500) -> ()  [unwired: 1 out]
          }
          frame #3 {
            n154 = property on="Current \nTemperature" class="DigNum (strict)"() -> ("Value"=w370:dbl)  [unwired: 2 in, 2 out]
            n155 = Path To String(path="Image file path \n(Do not add specify file extension - set to png)") -> (string=w365:string)
            n156 = Number To Fractional String(number=w370, precision (6)=i16 2 ("width (-)")) -> (F-format string=w367:string)  [unwired: 2 in]
            n157 = Concatenate Strings("_" ("string"), w367) -> (w364:string)
            n158 = Concatenate Strings(w365, w364) -> (w363:string)
            n159 = call <vilib>:"IMAQdx Grab2.vi"("error in"=w375, "Image In"=w374, "Session In"=w373) -> ("error out"=w376:errorcluster, "Image Out"=w371:T2, "Session Out"=w372:T5)  [unwired: 5 in, 1 out]
            n160 = Concatenate Strings(w363, ".png" ("string")) -> (w361:string)
            n161 = String To Path(string=w361) -> (path=w360:path)
            n162 = call-poly "IMAQ Write File 2"("File Path"=w360, "Image"=w371) -> ()  [unwired: 8 in, 2 out]
          }
          frame #4 {
            n163 = property on="ON/OFF" class="Bool (strict)"("Val(Sgnl)"=FALSE ("ON/OFF")) -> ()  [unwired: 2 in, 2 out]
          }
          frame #5 {
            n164 = local write "Record"(FALSE ("Record")) -> ()
          }
          frame #6 {
            n165 = property on="Action" class="LstBox (strict)"("Val(Sgnl)"=0 ("Value (Signaling)")) -> ()  [unwired: 2 in, 2 out]
          }
        }
      }
      frame 2 {
        n166 = flat-sequence {
          tunnel: w412 -> [w416]
          tunnel: w413 -> [w417]
          tunnel: w414 -> [w418]
          tunnel: [w418] -> w409
          tunnel: [w417] -> w408
          tunnel: [w416] -> w407
          tunnel: w409 -> [w432]
          tunnel: [w432] -> w406
          tunnel: w408 -> [w431]
          tunnel: [w431] -> w404
          tunnel: w407 -> [w430]
          tunnel: [w430] -> w402
          tunnel: [w427] -> w395
          tunnel: w406 -> [w436]
          tunnel: [w436] -> w405
          tunnel: w404 -> [w435]
          tunnel: [w435] -> w403
          tunnel: w402 -> [w434]
          tunnel: [w434] -> w401
          tunnel: [w433] -> w396
          tunnel: w395 -> [w433]
          tunnel: w405 -> [w438]
          tunnel: w403 -> [w439]
          tunnel: w401 -> [w440]
          tunnel: [w440] -> w400
          tunnel: [w439] -> w399
          tunnel: [w438] -> w398
          tunnel: [w437] -> w397
          tunnel: w396 -> [w437]
          tunnel: w400 -> [w447]
          tunnel: w399 -> [w446]
          tunnel: w398 -> [w445]
          tunnel: [w443] -> w394
          tunnel: [w444] -> w393
          tunnel: [w448] -> w392
          tunnel: w397 -> [w442]
          tunnel: w394 -> [w461]
          tunnel: [w461] -> w389
          tunnel: w393 -> [w460]
          tunnel: [w460] -> w391
          tunnel: w392 -> [w459]
          tunnel: w391 -> [w464]
          tunnel: [w464] -> w390
          tunnel: w389 -> [w463]
          tunnel: [w463] -> w388
          tunnel: w390 -> [w466]
          tunnel: w388 -> [w467]
          tunnel: [w467] -> w387
          tunnel: [w466] -> w386
          tunnel: [w469] -> w410
          tunnel: [w470] -> w411
          tunnel: w387 -> [w470]
          tunnel: w386 -> [w469]
          frame #0 {
            n167 = property on="ON/OFF" class="Bool (strict)"("Val(Sgnl)"=TRUE ("Value (Signaling)")) -> ()  [unwired: 2 in, 2 out]
          }
          frame #1 {
            n168 = property on="Frame Rate" class="DigNum (strict)"() -> ("Value"=w425:dbl)  [unwired: 2 in, 2 out]
            n169 = Number To Decimal String(number=w425, width (-)=i16 2) -> (decimal integer string=w420:string)
            n170 = Wait (ms)(milliseconds to wait=u32 500) -> ()  [unwired: 1 out]
            n171 = Concatenate Strings("File path for video", "_" ("string"), w420, "Hz.avi" ("string")) -> (w422:string)
            n172 = String To Path(string=w422) -> (path=w423:path)
            n173 = call "IMAQ AVI2 Create"("Codec"="Motion JPEG (NI Vision)", "Frames Per Second"=w425, "AVI Path"=w423) -> ("AVI Refnum"=w427:T11)  [unwired: 7 in, 1 out]
          }
          frame #2 {
          }
          frame #3 {
            n174 = property on="Trigger Laser" class="Bool (strict)"("Val(Sgnl)"=TRUE ("Value (Signaling)")) -> ()  [unwired: 2 in, 2 out]
          }
          frame #4 {
            n175 = while {
              tunnel: w446 -> [w456]
              shift-right: [w454] -> w444
              shift-left: w447 -> [w457]
              shift-right: [w453] -> w443
              shift-left: w445 -> [w455]
              shift-right: [w458] -> w448
              shift-left: w442 -> [w452]
              stop <- w450 stop-if-true
              n176 = call <vilib>:"IMAQdx Grab2.vi"("error in"=w457, "Image In"=w456, "Session In"=w455) -> ("error out"=w454:errorcluster, "Image Out"=w451:T2, "Session Out"=w453:T5)  [unwired: 5 in, 1 out]
              n177 = call "IMAQ AVI2 Write Frame"("Image"=w451, "AVI Refnum"=w452) -> ("AVI Refnum (duplicate)"=w458:T11)  [unwired: 7 in, 2 out]
              n178 = property on="Video" class="Bool (strict)"() -> ("Value"=w449:bool)  [unwired: 2 in, 2 out]
              n179 = Not(x=w449) -> (.not. x?=w450:bool)
            }
          }
          frame #5 {
            n180 = call "IMAQ AVI2 Close"("AVI Refnum"=w459) -> ()  [unwired: 10 in, 1 out]
          }
          frame #6 {
            n181 = property on="ON/OFF" class="Bool (strict)"("Val(Sgnl)"=FALSE ("Value (Signaling)")) -> ()  [unwired: 2 in, 2 out]
          }
          frame #7 {
            n182 = property on="Action" class="LstBox (strict)"("Val(Sgnl)"=0 ("Value (Signaling)")) -> ()  [unwired: 2 in, 2 out]
          }
          frame #8 {
            n183 = property on="Trigger Laser" class="Bool (strict)"("Val(Sgnl)"=FALSE ("Value (Signaling)")) -> ()  [unwired: 2 in, 2 out]
          }
        }
      }
    }
  }
  "error out" <- w54
  n184 = Initialize Array(0.0 ("element"), 1 ("dimension size")) -> (→"varLaplacian":dbl[])
  n185 = Initialize Array(0.0 ("element"), 1 ("dimension size")) -> (→"meanIntensity":dbl[])
  n186 = call <vilib>:"IMAQdx Close Camera.vi"("Session In"=w6) -> ()  [unwired: 10 in, 1 out]
  "steps" <- w3
  "displacement" <- w4
  "Direction" <- TRUE ("Clockwise/Counterclockwise?")
  "Turn" <- FALSE
